vi "Neuron_Layer.vi"(2 "b":T1, 3 "A_l-1":T1, 4 "W":T1, 5 "Activation":T2) -> (0 "A_l":T1, 1 "Z":T1)   [LabVIEW 2016]
uses:
  <vilib>/Analysis/Matrix/Datatypes/RealMatrix.ctl
  Enum_activations.ctl
  <vilib>/Analysis/Matrix/NI_Matrix.lvlib
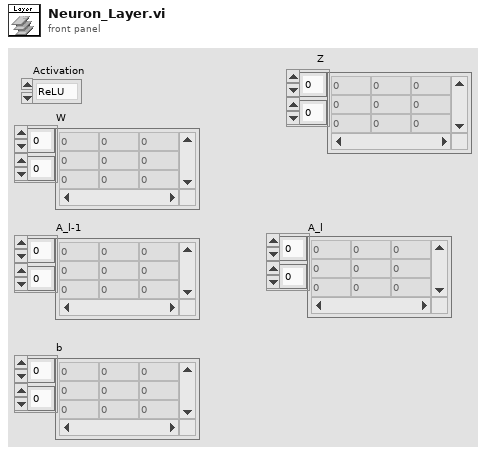
[diagram p1: front panel]
types:
  T1 = typedef "NI_Matrix.lvlib/RealMatrix.ctl" = dbl[][]
  T2 = typedef "Enum_activations.ctl" = enum16{"ReLU", "Sigmoid"}
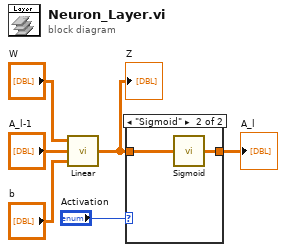
[diagram p0: block diagram]
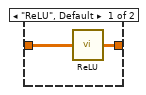
[diagram p2: hidden frame]
diagram:
  n1 = call "Linear.vi"("b"="b", "A"="A_l-1", "W"="W") -> ("Z"=w1:T1)
  "Z" <- w1
  n2 = case shown="\"Sigmoid\"" "Activation" {
    tunnel: w1 -> [w8 w10]
    tunnel: [w7 w9] -> w2
    frame "ReLU", Default {
      n3 = call "ReLU.vi"("Z"=w8) -> ("Relu"=w7:T1)
    }
    frame "Sigmoid" {
      n4 = call "Sigmoid.vi"("Z matrix"=w10) -> ("Sigmoid"=w9:T1)
    }
  }
  "A_l" <- w2
